vi "Set_Init_States_Manual.vi"(2 "register 2 (8-13)":T1=[FALSE, FALSE, FALSE, FALSE, FALSE, FALSE], 3 "register 1 (2-7)":T2, 8 "error in":errorcluster, 11 "Filename (ini)":string="Config_Ver_1\\pulse_sequence.ini") -> (0 "error out":errorcluster)   [LabVIEW 2021]
uses:
  Initial_States.ctl
  Channel_State.ctl
  Drivers/Arduino_Pulse_Generator/Configurate/Register_1.ctl
  Drivers/Arduino_Pulse_Generator/Configurate/Register_2.ctl
  <vilib>/Utility/config.llb/Write Key (Boolean).vi
  <vilib>/Utility/config.llb/NI_LVConfig.lvlib
panel:
  in  "Initial states":T3
  in  "End configuration":bool
  in  "Channel map filename (.ini)":string="channels_map_default.ini"
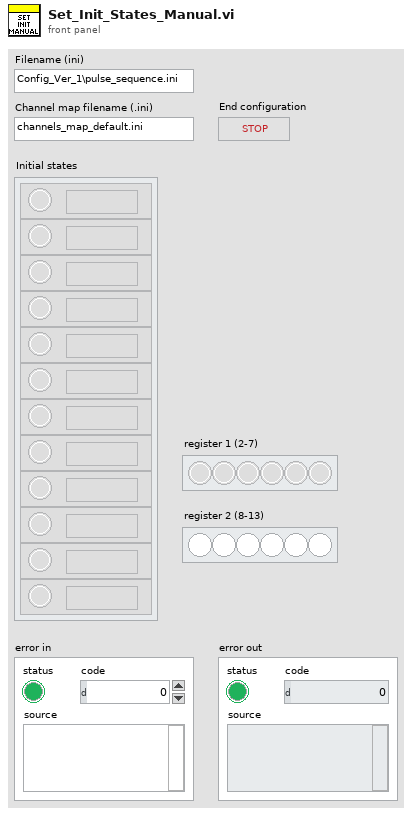
[diagram p1: front panel]
types:
  T1 = typedef "Register_2.ctl" = bool[]
  T2 = typedef "Register_1.ctl" = bool[]
  T3 = typedef "Initial_States.ctl" = T4[]
  T4 = typedef "Channel_State.ctl" = cluster{"state":bool, "chan name":string}
  T5 = typedef "Channels_Map.ctl" = T6[]
  T6 = typedef "Channel_Cluster.ctl" = cluster{"Channel name":string, "Channel":u8}
  T7 = typedef "NI_LVConfig.lvlib/Config Data RefNum.ctl" = refnum<k1>
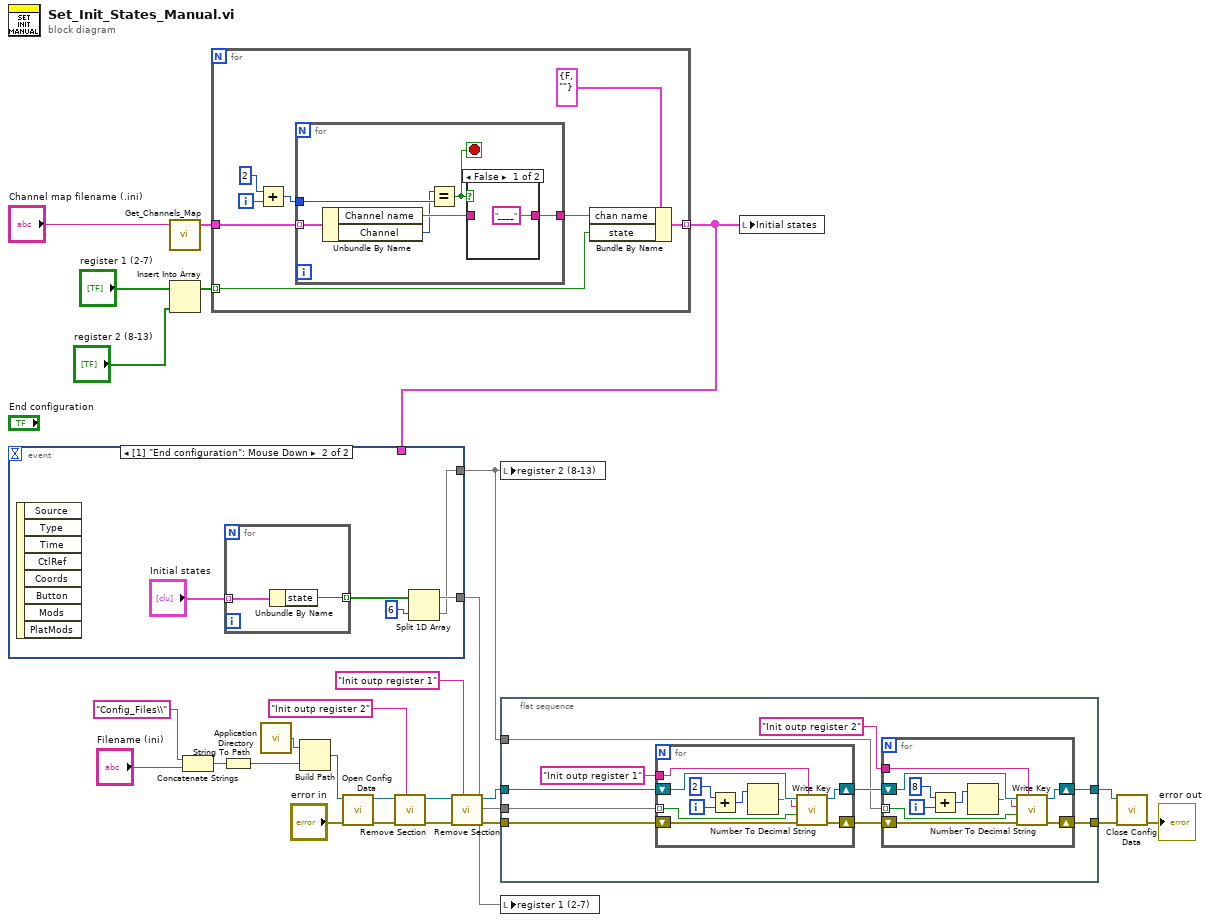
[diagram p0: block diagram]
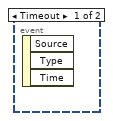
[diagram p3: hidden frame]
diagram:
  n1 = call "Get_Channels_Map.vi"("Filename (.ini)"="Channel map filename (.ini)") -> ("Channels Map"=w23:T5)  [unwired: 3 in, 1 out]
  n2 = Insert Into Array(array="register 1 (2-7)", new element="register 2 (8-13)") -> (w22:T2)  [unwired: 1 in]
  n3 = Concatenate Strings("Config_Files\\" ("string"), "Filename (ini)") -> (w17:string)
  n4 = for {
    tunnel: w23 -> [w31]
    tunnel: w22 -> [w33] mode=indexing
    tunnel: [w32] -> w1 mode=indexing
    i -> [w28]
    n5 = Add(x=2, y=w28) -> (x+y=w29:i32)
    n6 = for {
      tunnel: w31 -> [w40] mode=indexing
      tunnel: w29 -> [w39]
      tunnel: [w37] -> w30
      stop <- w38 stop-if-true
      n7 = Unbundle By Name(w40) -> ("Channel name"=w36:string, "Channel"=w35:u8)
      n8 = Equal?(x=w35, y=w39) -> (x = y?=w38:bool)
      n9 = case shown="False" w38 {
        tunnel: ["____" w42] -> w37
        tunnel: w36 -> [_ w42]
        frame False {
        }
        frame True {
        }
      }
    }
    n10 = Bundle By Name(cluster=T4 {"state"=FALSE, "chan name"=""} ("Chan state"), "chan name"=w30, "state"=w33) -> (w32:T4)
  }
  n11 = event shown="[1] \"End configuration\": Mouse Down" {
    selector: _ -> [_ _]
    dyn-events: _ -> [_ _]
    timeout: _ -> [_ _]
    tunnel: [_ w45] -> w11
    tunnel: [_ w44] -> w2
    tunnel: w1 -> [_ _]
    event Timeout {
      n12 = event-data() -> ()  [unwired: 1 in, 3 out]
    }
    event "End configuration": Mouse Down {
      n13 = event-data() -> ()  [unwired: 1 in, 8 out]
      n14 = for {
        tunnel: "Initial states" -> [w49] mode=indexing
        tunnel: [w48] -> w47 mode=indexing
        n15 = Unbundle By Name(w49) -> ("state"=w48:bool)
      }
      n16 = Split 1D Array(array=w47, index=6) -> (first subarray=w45:bool[], second subarray=w44:bool[])
    }
  }
  n17 = String To Path(string=w17) -> (path=w15:path)
  n18 = call <vilib>:"Application Directory.vi"() -> ("Application Directory"=w4:path)
  n19 = Build Path(base path=w4, name or relative path=w15) -> (appended path=w13:path)
  n20 = call <vilib>:"Open Config Data.vi"("error in (no error)"="error in", "configuration file path"=w13) -> ("error out"=w21:errorcluster, "refnum"=w20:T7)  [unwired: 7 in, 1 out]
  n21 = call <vilib>:"Remove Section.vi"("section"="Init outp register 2", "error in (no error)"=w21, "refnum"=w20) -> ("error out"=w18:errorcluster, "refnum out"=w19:T7)  [unwired: 6 in, 1 out]
  n22 = call <vilib>:"Remove Section.vi"("section"="Init outp register 1", "error in (no error)"=w18, "refnum"=w19) -> ("error out"=w3:errorcluster, "refnum out"=w12:T7)  [unwired: 6 in, 1 out]
  n23 = local write "register 2 (8-13)"(w2) -> ()
  n24 = flat-sequence {
    tunnel: w3 -> [w59]
    tunnel: w12 -> [w58]
    tunnel: [w53] -> w8
    tunnel: [w52] -> w9
    tunnel: w2 -> [w51]
    tunnel: w11 -> [w50]
    frame #0 {
      n25 = for {
        tunnel: w50 -> [w73] mode=indexing
        shift-right: [w78] -> w56
        shift-left: w59 -> [w76]
        shift-right: [w77] -> w55
        shift-left: w58 -> [w79]
        tunnel: "Init outp register 1" ("section") -> [w70]
        i -> [w75]
        n26 = Add(x=2, y=w75) -> (x+y=w72:i32)
        n27 = Number To Decimal String(number=w72) -> (decimal integer string=w71:string)  [unwired: 1 in]
        n28 = call-poly <vilib>:"Write Key.vi"("section"=w70, "error in (no error)"=w76, "value"=w73, "key"=w71, "refnum"=w79) -> ("error out"=w78:errorcluster, "refnum out"=w77:T7)  [unwired: 4 in, 1 out]
      }
      n29 = for {
        tunnel: w51 -> [w63] mode=indexing
        shift-right: [w68] -> w53
        shift-left: w56 -> [w66]
        shift-right: [w67] -> w52
        shift-left: w55 -> [w69]
        tunnel: "Init outp register 2" ("section") -> [w60]
        i -> [w65]
        n30 = Add(x=8, y=w65) -> (x+y=w62:i32)
        n31 = Number To Decimal String(number=w62) -> (decimal integer string=w61:string)  [unwired: 1 in]
        n32 = call-poly <vilib>:"Write Key.vi"("section"=w60, "error in (no error)"=w66, "value"=w63, "key"=w61, "refnum"=w69) -> ("error out"=w68:errorcluster, "refnum out"=w67:T7)  [unwired: 4 in, 1 out]
      }
    }
  }
  n33 = local write "register 1 (2-7)"(w11) -> ()
  n34 = local write "Initial states"(w1) -> ()
  n35 = call <vilib>:"Close Config Data.vi"("error in (no error)"=w8, "refnum"=w9) -> ("error out"=→"error out":errorcluster)  [unwired: 8 in, 1 out]
